vi "sort2DArrayAscDesc.vi"(4 "Descending? (T)":bool=TRUE, 5 "2D Array":i32[][](array[numeric])) -> (1 "sorted 2D array":i32[][](array[numeric]))   [LabVIEW 2019]
uses:
  fac411f6-ba32-440e-a36d-a0029fd44cdc.vi
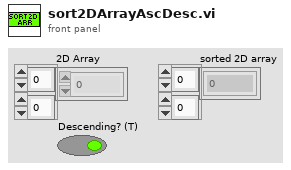
[diagram p1: front panel]
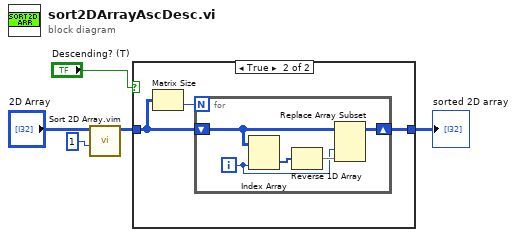
[diagram p0: block diagram]
diagram:
  n1 = call "Sort 2D Array.vim"("index"=1, "2D array"="2D Array") -> ("sorted 2D array"=w3:i32[][])  [unwired: 8 in, 1 out]
  n2 = case shown="True" "Descending? (T)" {
    tunnel: [w6 w9] -> w4
    tunnel: w3 -> [w6 w7]
    frame False {
    }
    frame True {
      n3 = Matrix Size(0:w7) -> (2:w8:i32)  [unwired: 1 out]
      n4 = for {
        N: w8 -> [_]
        shift-right: [w12] -> w9
        shift-left: w7 -> [w13]
        i -> [w10]
        n5 = Index Array(array=w13, index (col)=w10) -> (element=w14:i32[])  [unwired: 1 in]
        n6 = Reverse 1D Array(array=w14) -> (reversed array=w11:i32[])
        n7 = Replace Array Subset(array=w13, new element=w11, index (col)=w10) -> (w12:i32[][])  [unwired: 1 in]
      }
    }
  }
  "sorted 2D array" <- w4
